vi "Actor Core.vi"(8 "error in":errorcluster, 11 "Nested in":refnum<class "Network Test.lvclass">) -> (0 "error out":errorcluster, 3 "Actor out":refnum<class "Actor.lvclass">)   [LabVIEW 2017, in "Network Test.lvlib" / "Network Test.lvclass"]
doc: "(<B>Filename</B>: Actor Framework.lvlib:Actor.lvclass:Actor Core.vi)\n\nReceives messages to the actor, reacts to them, and initiates any error handling that may shut the actor down.\n\nDescendant classes may override this VI to append parallel tasks for the actor to complete while it handles messages. Overrides use the Call Parent Method node."
uses:
  Network Test.lvclass
  C:/Program Files (x86)/National Instruments/LabVIEW 2017/vi.lib/ActorFramework/Actor/Actor.lvclass
  <vilib>/ActorFramework/Actor/Actor.lvclass
  Network Test Helper Loop States.ctl
  <vilib>/ActorFramework/Message Enqueuer/Message Enqueuer.lvclass
  Ping Test Configuration.ctl
  Network Test.lvclass/Network Test.ctl
  <vilib>/ActorFramework/Actor/Actor.lvclass/Actor.ctl
  <vilib>/ActorFramework/Message Enqueuer/Message Enqueuer.lvclass/Message Enqueuer.ctl
  Test/Test Messages/Update Test Progress Msg/Update Test Progress Msg.lvclass/Update Test Progress Msg.ctl
  Network Test Messages/Ping N Times Msg/Ping N Times Msg.lvclass/Ping N Times Msg.ctl
  <vilib>/ActorFramework/Message Enqueuer/Init from Existing Queue.vi
  <vilib>/ActorFramework/Message Enqueuer/Enqueue.vi
  Test/Test Messages/Update Test Progress Msg/Update Test Progress Msg.lvclass
  C:/Program Files (x86)/National Instruments/LabVIEW 2017/vi.lib/ActorFramework/Message/Message.lvclass
  Network Test Messages/Ping N Times Msg/Ping N Times Msg.lvclass
  <vilib>/ActorFramework/Message Priority Queue/Priority Enqueue.vi
  Test/Test/Test.lvclass
  Network Test.lvlib
panel:
  out "Packet Returned":dbl
  out "Ping Test":i32[](listbox)
  out "Ping Status":string
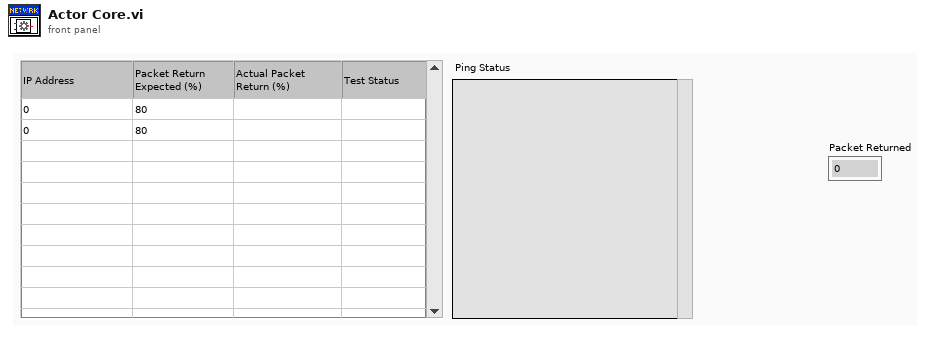
[diagram p1: front panel]
types:
  T1 = typedef "Network Test.lvlib/Ping Test Configuration.ctl" = cluster{"IP/Address":string, "PacketSize":i32, "timeout":i32, "Packet Count":i32, "Min Expected Packed Return %":dbl, "Ping Result":cluster{"Result?":bool, "Actual Packet Return %":dbl}}
  T2 = cluster{"VI Name":string, "Self Enqueuer":refnum<class "Message Enqueuer.lvclass">, "Ping Test Configurations":T1[]}
  T3 = typedef "Network Test.lvlib/Network Test Helper Loop States.ctl" = enum16{"Poll", "Init", "Update UI", "Read Test Case Data", "Send Ping Request", "Update Result", "Error", "Exit"}
  T4 = cluster{"Stop":refnum<user-event>, "Packet Returned":refnum<user-event>, "Ping Status":refnum<user-event>, "Ping Test Result":refnum<user-event>, "Ping Test":refnum<user-event>}
  T5 = typedef "Paths.ctl" = cluster{"Data Directory":path, "Test Config Dir":path, "Error Logs":path, "Event Logs":path, "Settings.Json":path, "Reports Directory":path}
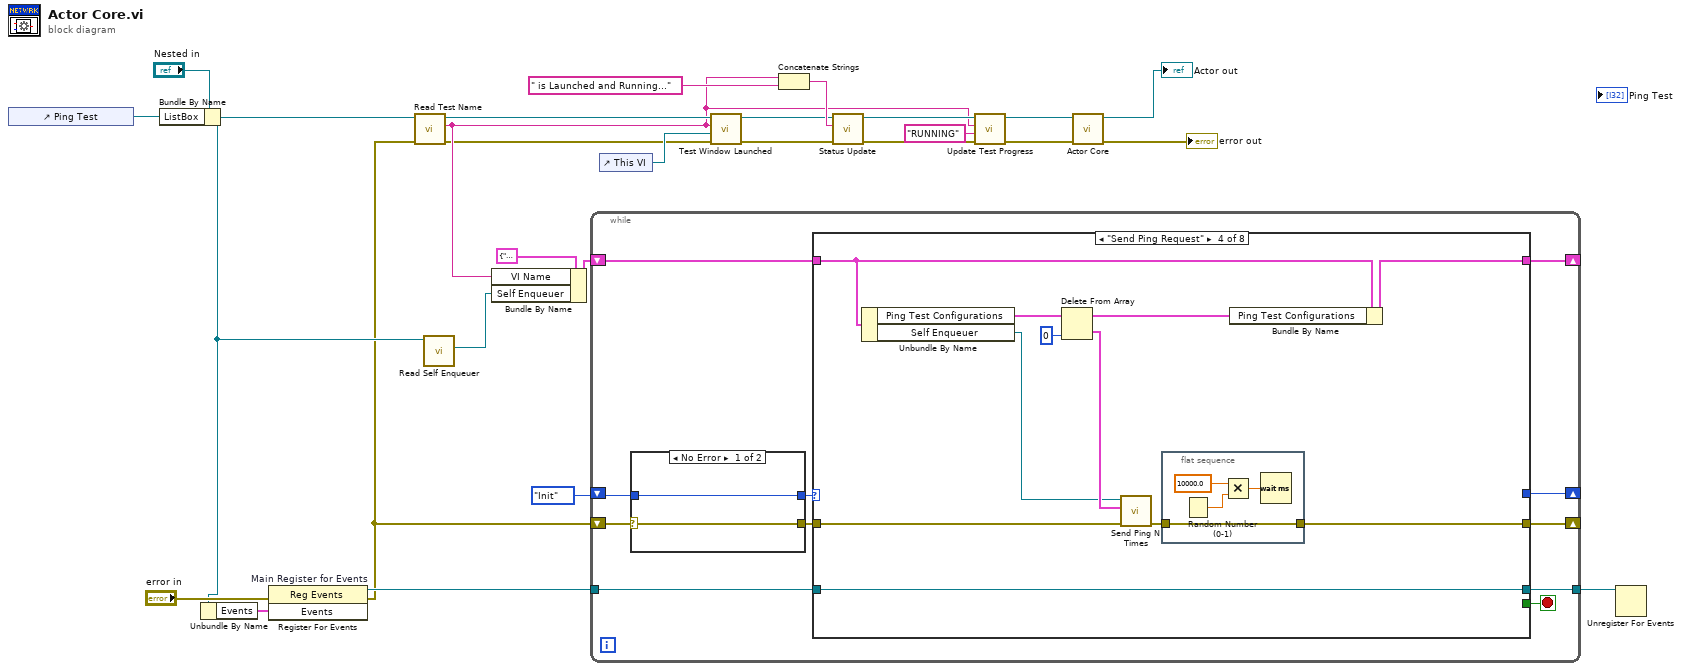
[diagram p0: block diagram]
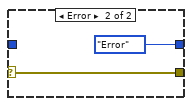
[diagram p2: hidden frame]
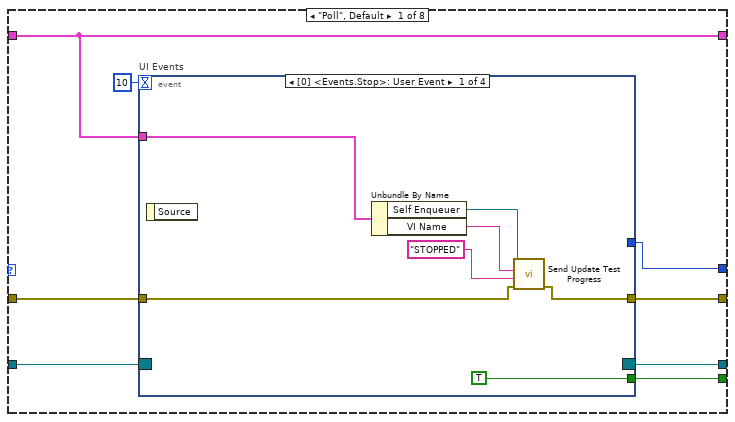
[diagram p3: hidden frame]
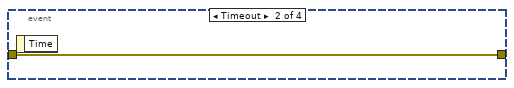
[diagram p4: hidden frame]
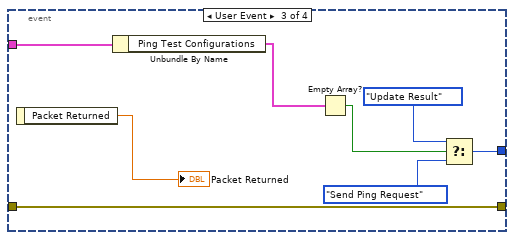
[diagram p5: hidden frame]
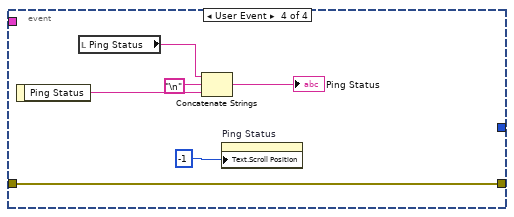
[diagram p6: hidden frame]
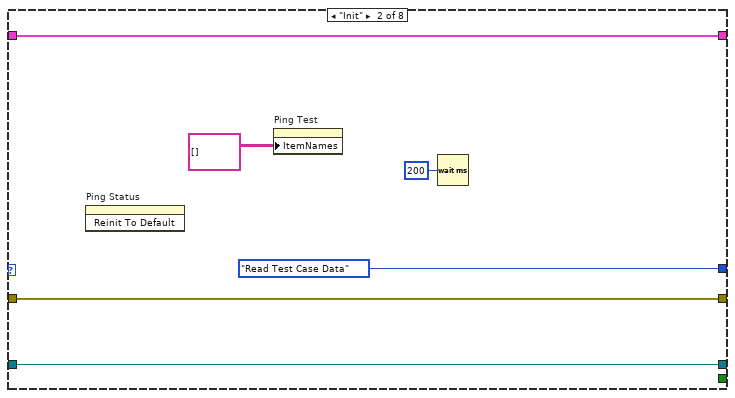
[diagram p7: hidden frame]
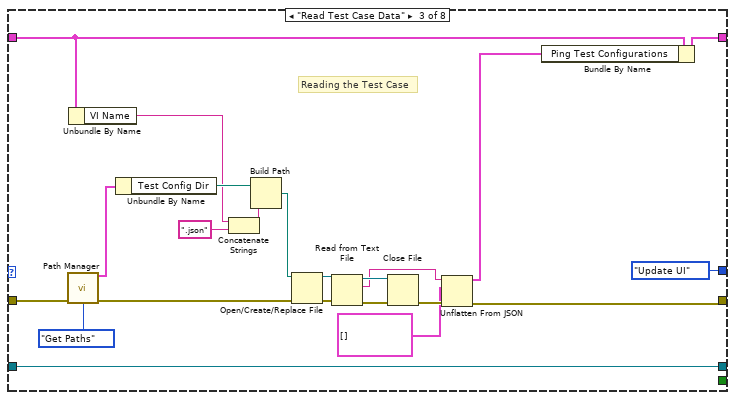
[diagram p8: hidden frame]
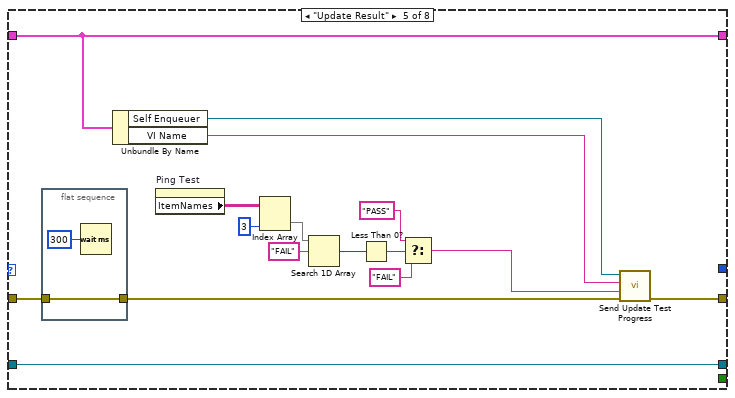
[diagram p9: hidden frame]
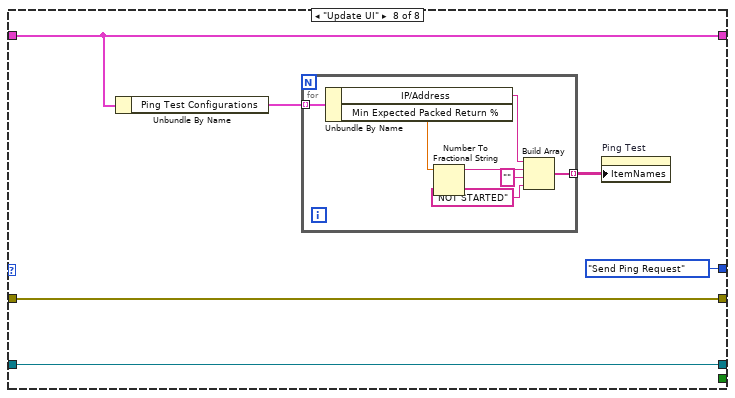
[diagram p12: hidden frame]
diagram:
  n1 = control-ref of="Ping Test"() -> (w14:refnum<vi>)
  n2 = Bundle By Name(cluster="Nested in", "ListBox"=w14) -> (w13:refnum<class "Network Test.lvclass">)
  n3 = Unbundle By Name(w13) -> ("Events"=w24:T4)
  n4 = register-events "Main Register for Events"(error in="error in", w24) -> (reference out=w25:refnum<event-registration>, error out=w3:errorcluster)  [unwired: 1 in]
  n5 = call-dynamic "Read Test Name.vi"("error in (no error)"=w3, "Test in"=w13) -> ("error out"=w2:errorcluster, "Test Name"=w4:string, "Test out"=w12:refnum<class "Network Test.lvclass">)  [unwired: 7 in]
  n6 = call <vilib>:"Read Self Enqueuer.vi"("Actor"=w13) -> ("Self Enqueuer"=w1:refnum<class "Message Enqueuer.lvclass">)  [unwired: 10 in]
  n7 = Bundle By Name(cluster=T2 {"VI Name"="", "Self Enqueuer"=refnum, "Ping Test Configurations"=[]}, "VI Name"=w4, "Self Enqueuer"=w1) -> (w5:T2)
  n8 = while {
    tunnel: w25 -> [w38]
    tunnel: [w36] -> w23
    shift-right: [w31] -> _
    shift-left: w3 -> [w35]
    shift-right: [w30] -> _
    shift-left: Network_Test_Helper_Loop_States."Init" -> [w34]
    shift-right: [w28] -> _
    shift-left: w5 -> [w29]
    stop <- w37 stop-if-true
    n9 = case shown="No Error" w35 {
      selector: w35 -> [w40 w41]
      tunnel: w34 -> [w39 _]
      tunnel: [w40 w41] -> w32
      tunnel: [w39 Network_Test_Helper_Loop_States."Error"] -> w33
      frame No Error {
      }
      frame Error {
      }
    }
    n10 = case shown="\"Send Ping Request\"" w33 {
      tunnel: w38 -> [w50 w78 w100 w111 w131 w135 w138 w145]
      tunnel: [w49 _ _ _ _ _ _ _] -> w37
      tunnel: [w48 w78 w100 w111 w131 w135 w138 w145] -> w36
      tunnel: w32 -> [w46 w77 w89 w110 w117 w136 w139 w144]
      tunnel: [w45 w77 w92 w101 w128 w136 w139 w144] -> w31
      tunnel: [w43 Network_Test_Helper_Loop_States."Read Test Case Data" Network_Test_Helper_Loop_States."Update UI" _ _ _ _ Network_Test_Helper_Loop_States."Send Ping Request"] -> w30
      tunnel: w29 -> [w44 w75 w81 w109 w130 w134 w137 w143]
      tunnel: [w44 w75 w91 w108 w130 w134 w137 w143] -> w28
      frame "Poll", Default {
        n11 = event "UI Events" shown="[0] <Events.Stop>: User Event" {
          selector: w50 -> [_ _ _ _]
          dyn-events: [_ _ _ _] -> w48
          timeout: 10 -> [_ _ _ _]
          tunnel: [TRUE _ _ _] -> w49
          tunnel: w46 -> [w53 w58 w65 w70]
          tunnel: [w52 w58 w65 w70] -> w45
          tunnel: w44 -> [w51 _ w59 _]
          tunnel: [_ _ w60 _] -> w43
          event User Event {
            n12 = event-data() -> ()  [unwired: 1 in, 1 out]
            n13 = Unbundle By Name(w51) -> ("Self Enqueuer"=w54:refnum<class "Message Enqueuer.lvclass">, "VI Name"=w55:string)
            n14 = call "Send Update Test Progress.vi"("error in (no error)"=w53, "State"="STOPPED", "Test Name"=w55, "Message Enqueuer"=w54) -> ("error out"=w52:errorcluster)  [unwired: 6 in, 1 out]
          }
          event Timeout {
            n15 = event-data() -> ()  [unwired: 1 in, 1 out]
          }
          event User Event {
            n16 = event-data() -> ("Packet Returned"=→"Packet Returned":dbl)  [unwired: 1 in]
            n17 = Unbundle By Name(w59) -> ("Ping Test Configurations"=w64:T1[])
            n18 = Empty Array?(array=w64) -> (empty?=w63:bool)
            n19 = Select(t=Network_Test_Helper_Loop_States."Update Result", s=w63, f=Network_Test_Helper_Loop_States."Send Ping Request") -> (s? t:f=w60:T3)
          }
          event User Event {
            n20 = event-data() -> ("Ping Status"=w71:string)  [unwired: 1 in]
            n21 = local read "Ping Status"() -> (w68:string)
            n22 = Concatenate Strings(w68, "\n", w71) -> (→"Ping Status":string)
            n23 = property on="Ping Status" class="Str"("Text.Scroll Position"=-1) -> ()  [unwired: 2 in, 2 out]
          }
        }
      }
      frame "Init" {
        n24 = invoke on="Ping Status" class="Str" method="Reinit To Default"() -> ()  [unwired: 3 in, 3 out]
        n25 = property on="Ping Test" class="MCListbox (strict)"("ItemNames"=string[][] [] ("Item Names")) -> ()  [unwired: 2 in, 2 out]
        n26 = Wait (ms)(milliseconds to wait=u32 200) -> ()  [unwired: 1 out]
      }
      frame "Read Test Case Data" {
        # "Reading the Test Case"
        n27 = call "Path Manager.vi"("Error in (no error)"=w89, "Options"=enum16{"Get Paths", "Init Paths"}."Get Paths") -> ("Cluster"=w86:T5, "Error out"=w88:errorcluster)  [unwired: 12 in]
        n28 = Unbundle By Name(w81) -> ("VI Name"=w80:string)
        n29 = Unbundle By Name(w86) -> ("Test Config Dir"=w85:path)
        n30 = Concatenate Strings(w80, ".json" ("string")) -> (w84:string)
        n31 = Build Path(base path=w85, name or relative path=w84) -> (appended path=w82:path)
        n32 = Open/Create/Replace File(file path (use dialog)=w82, error in=w88) -> (refnum out=w99:refnum<file>, error out=w96:errorcluster)  [unwired: 4 in, 1 out]
        n33 = Read from Text File(file (use dialog)=w99, error in=w96) -> (refnum out=w97:refnum<file>, text=w93:string, error out=w98:errorcluster)  [unwired: 2 in, 1 out]
        n34 = Close File(refnum=w97, error in=w98) -> (error out=w95:errorcluster)  [unwired: 1 out]
        n35 = Unflatten From JSON(JSON string=w93, type and defaults=T1[] [] ("Array"), error in (no error)=w95) -> (value=w90:T1[], error out=w92:errorcluster)  [unwired: 4 in]
        n36 = Bundle By Name(cluster=w81, "Ping Test Configurations"=w90) -> (w91:T2)
      }
      frame "Send Ping Request" {
        n37 = Unbundle By Name(w109) -> ("Ping Test Configurations"=w107:T1[], "Self Enqueuer"=w103:refnum<class "Message Enqueuer.lvclass">)
        n38 = Delete From Array(array=w107, index=0) -> (deleted portion=w104:T1, array with subset deleted=w102:T1[])  [unwired: 1 in]
        n39 = call "Send Ping N Times.vi"("error in (no error)"=w110, "Ping Test"=w104, "Message Enqueuer"=w103) -> ("error out"=w105:errorcluster)  [unwired: 7 in, 1 out]
        n40 = flat-sequence {
          tunnel: w105 -> [w115]
          tunnel: [w115] -> w101
          frame #0 {
            n41 = Random Number (0-1)() -> (number: 0 to 1=w114:dbl)
            n42 = Multiply(x=10000.0, y=w114) -> (x*y=w112:dbl)
            n43 = Wait (ms)(milliseconds to wait=w112) -> ()  [unwired: 1 out]
          }
        }
        n44 = Bundle By Name(cluster=w109, "Ping Test Configurations"=w102) -> (w108:T2)
      }
      frame "Update Result" {
        n45 = flat-sequence {
          tunnel: w117 -> [w133]
          tunnel: [w133] -> w116
          frame #0 {
            n46 = Wait (ms)(milliseconds to wait=u32 300) -> ()  [unwired: 1 out]
          }
        }
        n47 = Unbundle By Name(w130) -> ("Self Enqueuer"=w127:refnum<class "Message Enqueuer.lvclass">, "VI Name"=w129:string)
        n48 = property on="Ping Test" class="MCListbox (strict)"() -> ("ItemNames"=w126:string[][])  [unwired: 2 in, 2 out]
        n49 = Index Array(array=w126, index (col)=3 ("disabled index (col)")) -> (element=w124:string[])  [unwired: 1 in]
        n50 = Search 1D Array(1D array=w124, element="FAIL") -> (index of element=w122:i32)  [unwired: 1 in]
        n51 = Less Than 0?(x=w122) -> (x < 0?=w121:bool)
        n52 = Select(t="PASS" ("element"), s=w121, f="FAIL" ("element")) -> (s? t:f=w118:string)
        n53 = call "Send Update Test Progress.vi"("error in (no error)"=w116, "State"=w118, "Test Name"=w129, "Message Enqueuer"=w127) -> ("error out"=w128:errorcluster)  [unwired: 6 in, 1 out]
      }
      frame "Error" {
      }
      frame "Exit" {
      }
      frame "Update UI" {
        n54 = Unbundle By Name(w143) -> ("Ping Test Configurations"=w142:T1[])
        n55 = for {
          tunnel: w142 -> [w152] mode=indexing
          tunnel: [w146] -> w141 mode=indexing
          n56 = Unbundle By Name(w152) -> ("IP/Address"=w151:string, "Min Expected Packed Return %"=w150:dbl)
          n57 = Number To Fractional String(number=w150) -> (F-format string=w149:string)  [unwired: 3 in]
          n58 = Build Array(w151, w149, "" ("element"), "NOT STARTED" ("element")) -> (w146:string[])
        }
        n59 = property on="Ping Test" class="MCListbox (strict)"("ItemNames"=w141) -> ()  [unwired: 2 in, 2 out]
      }
    }
  }
  n60 = control-ref of="This VI"() -> (w20:refnum<vi>)
  n61 = call-dynamic "Test Window Launched.vi"("error in (no error)"=w2, "VI Refnum"=w20, "Window Name"=w4, "Test in"=w12) -> ("error out"=w18:errorcluster, "Test out"=w15:refnum<class "Network Test.lvclass">)  [unwired: 6 in]
  n62 = Concatenate Strings(w4, " is Launched and Running..." ("Window Name")) -> (w16:string)
  n63 = call-dynamic "Status Update.vi"("error in (no error)"=w18, "Status"=w16, "Network Test in"=w15) -> ("error out"=w11:errorcluster, "Network Test out"=w9:refnum<class "Network Test.lvclass">)  [unwired: 7 in]
  n64 = call-dynamic "Update Test Progress.vi"("error in (no error)"=w11, "State"="RUNNING", "Test Name"=w4, "Test in"=w9) -> ("error out"=w10:errorcluster, "Test out"=w8:refnum<class "Network Test.lvclass">)  [unwired: 6 in]
  n65 = call-parent "Actor Core.vi"("error in"=w10, "Actor in"=w8) -> ("error out"=→"error out":errorcluster, "Actor out"=→"Actor out":refnum<class "Actor.lvclass">)  [unwired: 8 in]
  n66 = Unregister For Events(event registration refnum=w23) -> ()  [unwired: 1 in, 1 out]
